vi "Cockpit UDP receiver v2.vi"() -> ()   [LabVIEW 2010]
panel:
  out "Waveform Chart 4":sgl(graph)
  out "Waveform Chart 3":sgl(graph)
  out "Waveform Chart 2":sgl(graph)
  out "Waveform Chart":sgl(graph)
  out "right_pedal":bool
  out "left_pedal":bool
  out "up_pedal":bool
  out "gripper":sgl
  out "down_pedal":sgl format="%.2f"
  out "rotation":sgl
  out "d 3":sgl
  out "theta 2":sgl
  out "length":i32
  out "data out":string
  out "theta 1":sgl
  in  "stop":bool
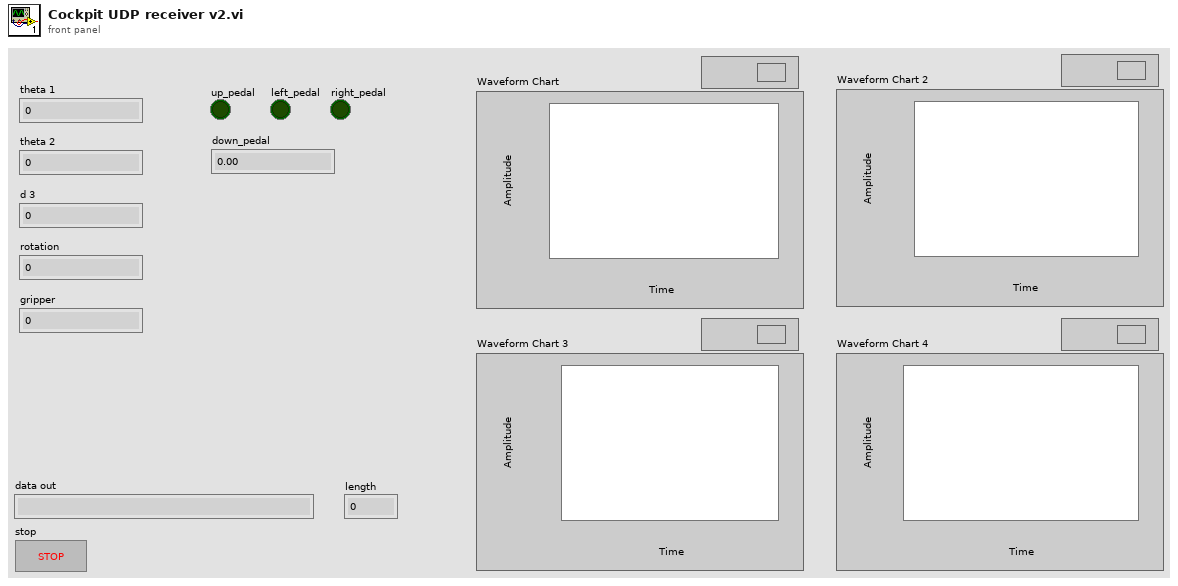
[diagram p1: front panel]
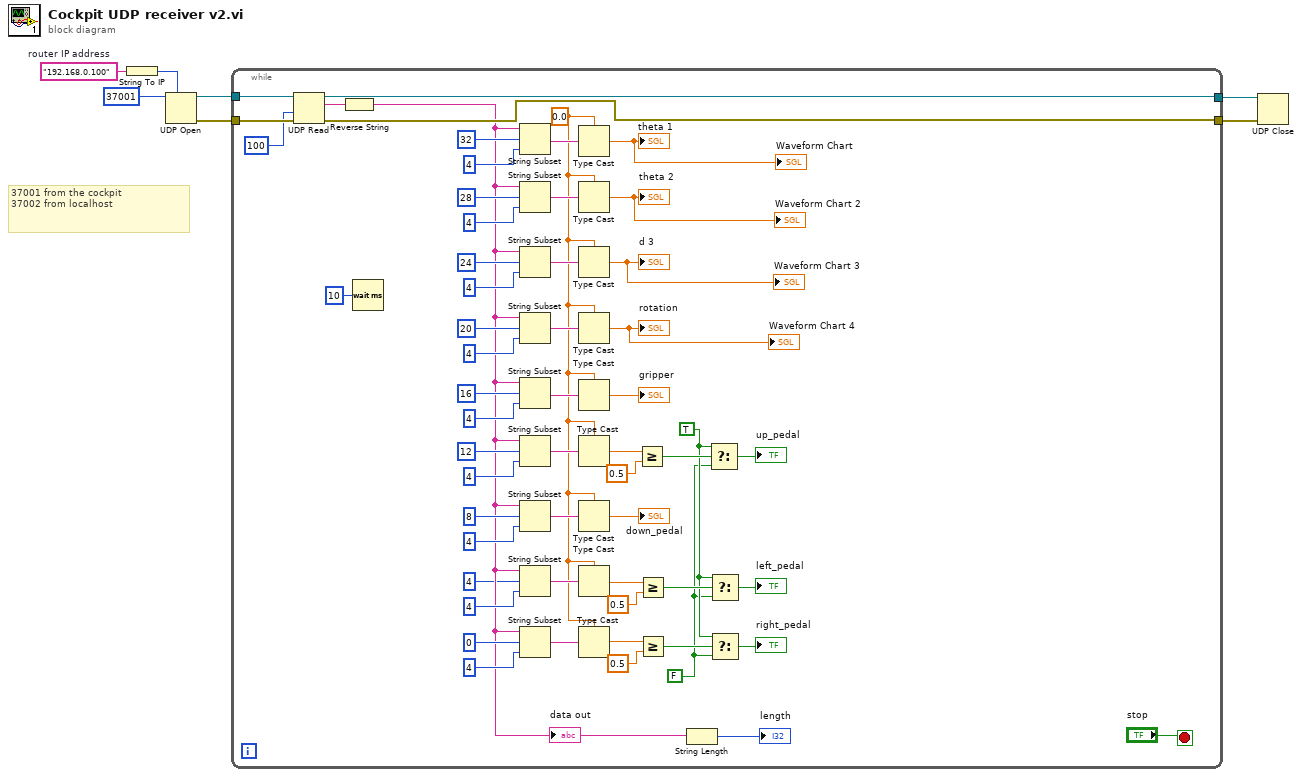
[diagram p0: block diagram]
diagram:
  w2 = "192.168.0.100"  # router IP address
  # "37001 from the cockpit\n37002 from localhost"
  n1 = String To IP(1:w2) -> (0:w1:u32)
  n2 = UDP Open(7:w1, 11:u16 37001 ("port")) -> (port=w6:refnum<k16>, 0:w4:errorcluster)  [unwired: 3 in, 1 out]
  n3 = while {
    tunnel: w6 -> [w65]
    tunnel: [w63] -> w5
    tunnel: w4 -> [w34]
    tunnel: [w33] -> w3
    stop <- "stop" stop-if-true
    w18 = FALSE
    w19 = TRUE
    w29 = sgl 0.0
    n4 = UDP Read(connection ID=w65, timeout ms (25000)=100, 8:w34) -> (data out=w32:string, error out=w33:errorcluster, 3:w63:refnum<k16>)  [unwired: 1 in, 2 out]
    n5 = Reverse String(1:w32) -> (0:w31:string)
    "data out" <- w31
    n6 = Wait (ms)(milliseconds to wait=u32 10) -> ()  [unwired: 1 out]
    n7 = String Subset(string=w31, offset (0)=32, length (rest)=4 ("offset (0)")) -> (substring=w60:string)
    n8 = String Subset(string=w31, offset (0)=28, length (rest)=4 ("offset (0)")) -> (substring=w52:string)
    n9 = String Subset(string=w31, offset (0)=24, length (rest)=4 ("offset (0)")) -> (substring=w51:string)
    n10 = String Subset(string=w31, offset (0)=20, length (rest)=4 ("offset (0)")) -> (substring=w50:string)
    n11 = String Subset(string=w31, offset (0)=16, length (rest)=4 ("offset (0)")) -> (substring=w40:string)
    n12 = String Subset(string=w31, offset (0)=12, length (rest)=4 ("offset (0)")) -> (substring=w47:string)
    n13 = String Subset(string=w31, offset (0)=8, length (rest)=4 ("offset (0)")) -> (substring=w48:string)
    n14 = String Subset(string=w31, offset (0)=4, length (rest)=4 ("offset (0)")) -> (substring=w49:string)
    n15 = String Subset(string=w31, offset (0)=0, length (rest)=4 ("offset (0)")) -> (substring=w35:string)
    n16 = Type Cast(type=w29, x=w60) -> (*(type *) &x=→"theta 1" →"Waveform Chart":sgl)
    n17 = Type Cast(type=w29, x=w52) -> (*(type *) &x=→"theta 2" →"Waveform Chart 2":sgl)
    n18 = Type Cast(type=w29, x=w51) -> (*(type *) &x=→"d 3" →"Waveform Chart 3":sgl)
    n19 = Type Cast(type=w29, x=w50) -> (*(type *) &x=→"rotation" →"Waveform Chart 4":sgl)
    n20 = Type Cast(type=w29, x=w40) -> (*(type *) &x=→"gripper":sgl)
    n21 = Type Cast(type=w29, x=w47) -> (*(type *) &x=w26:sgl)
    n22 = Type Cast(type=w29, x=w48) -> (*(type *) &x=→"down_pedal":sgl)
    n23 = Type Cast(type=w29, x=w49) -> (*(type *) &x=w20:sgl)
    n24 = Type Cast(type=w29, x=w35) -> (*(type *) &x=w21:sgl)
    n25 = Greater Or Equal?(x=w26, y=sgl 0.5) -> (x >= y?=w28:bool)
    n26 = Greater Or Equal?(x=w20, y=sgl 0.5) -> (x >= y?=w24:bool)
    n27 = Greater Or Equal?(x=w21, y=sgl 0.5) -> (x >= y?=w23:bool)
    n28 = String Length(string=w31) -> (length=→"length":i32)
    n29 = Select(t=w19, s=w28, f=w18) -> (s? t:f=→"up_pedal":bool)
    n30 = Select(t=w19, s=w24, f=w18) -> (s? t:f=→"left_pedal":bool)
    n31 = Select(t=w19, s=w23, f=w18) -> (s? t:f=→"right_pedal":bool)
  }
  n32 = UDP Close(connection ID=w5, 8:w3) -> ()  [unwired: 2 out]
